vi "YOKOGAWA OPTIONS.vi"(8 "Error In":errorcluster, 11 "VISA resource name":refnum<visa-resource-name>) -> (0 "Error Out":errorcluster, 2 "Yokogawa Options":T1, 3 "VISA resource name out":refnum<visa-resource-name>)   [LabVIEW 2016]
uses:
  Type Definitions/YOKOGAWA Options.ctl
  <vilib>/Utility/error.llb/whitespace.ctl
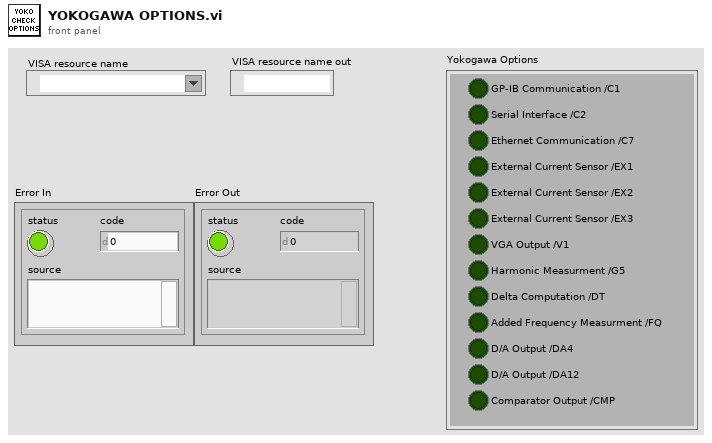
[diagram p1: front panel]
types:
  T1 = typedef "YOKOGAWA Options.ctl" = cluster{"GP-IB Communication /C1":bool, "Ethernet Communication /C7":bool, "External Current Sensor /EX1":bool, "External Current Sensor /EX2":bool, "External Current Sensor /EX3":bool, "VGA Output /V1":bool, "Harmonic Measurment /G5":bool, "Delta Computation /DT":bool, "Added Frequency Measurment /FQ":bool, "Serial Interface /C2":bool, "D/A Output /DA4":bool, "D/A Output /DA12":bool, "Comparator Output /CMP":bool}
  T2 = typedef "whitespace.ctl" = u16
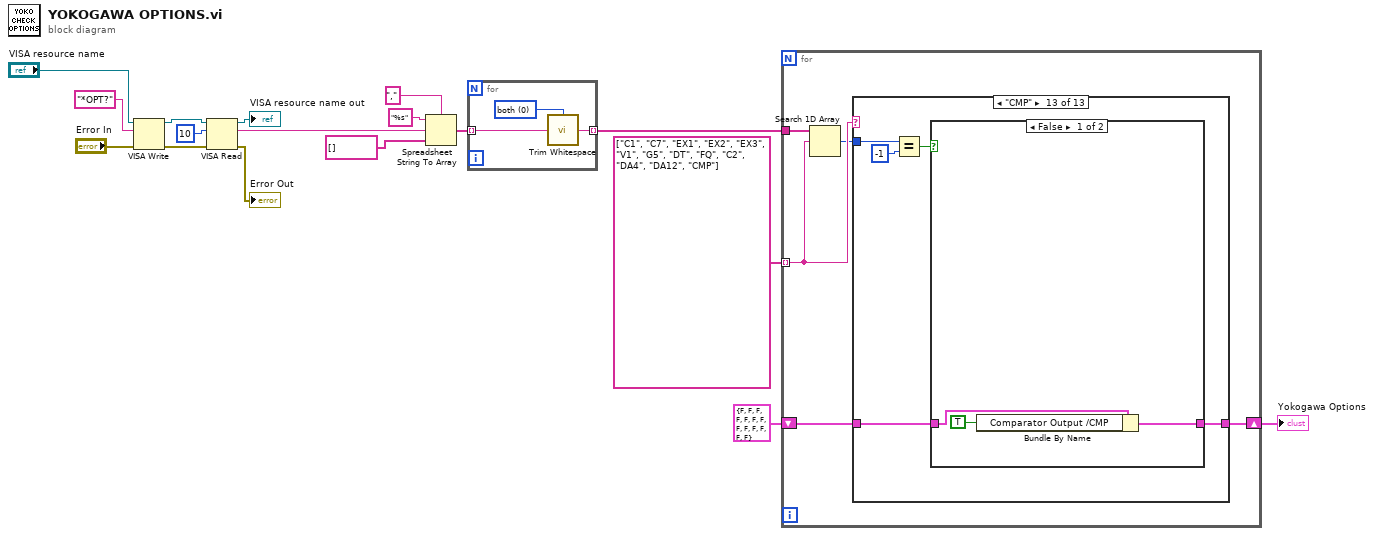
[diagram p0: block diagram]
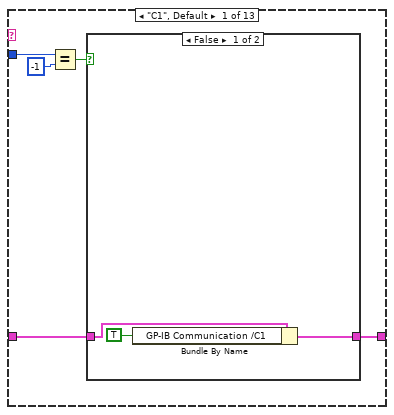
[diagram p2: hidden frame]
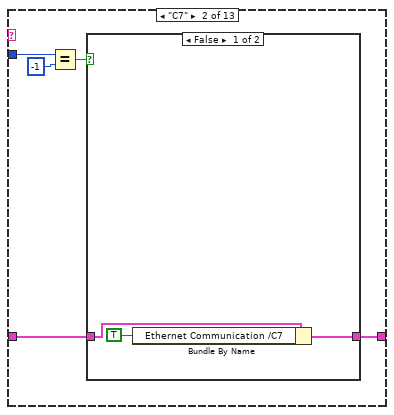
[diagram p4: hidden frame]
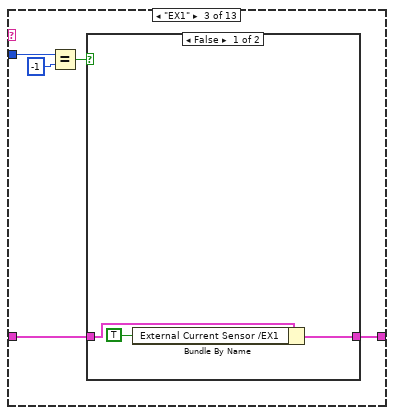
[diagram p6: hidden frame]
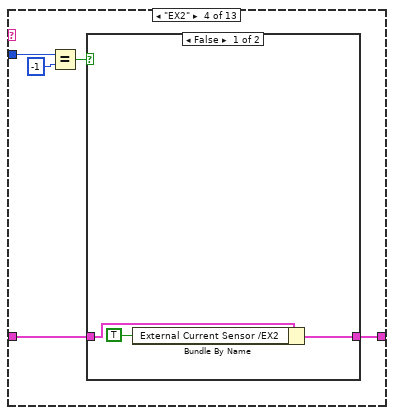
[diagram p8: hidden frame]
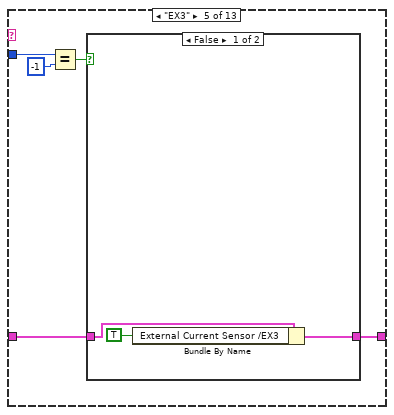
[diagram p10: hidden frame]
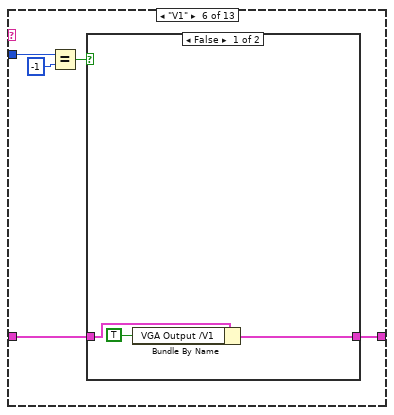
[diagram p12: hidden frame]
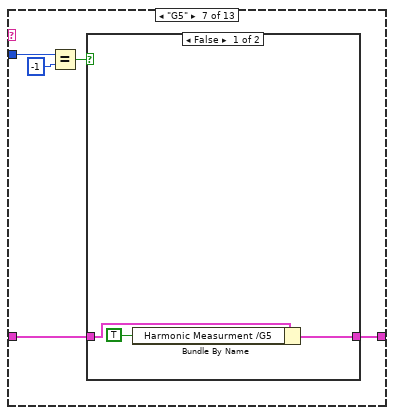
[diagram p14: hidden frame]
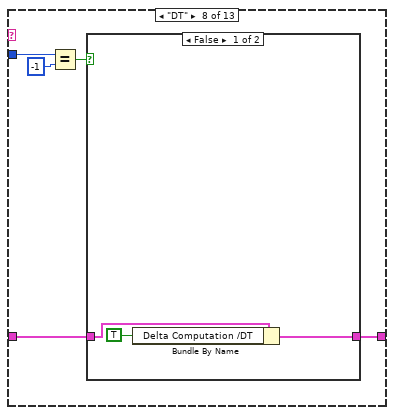
[diagram p16: hidden frame]
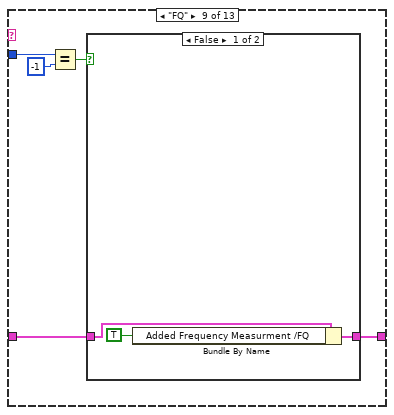
[diagram p18: hidden frame]
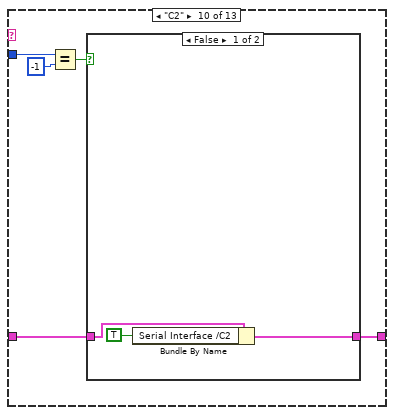
[diagram p20: hidden frame]
diagram:
  n1 = VISA Write(VISA resource name="VISA resource name", write buffer="*OPT?", error in (no error)="Error In") -> (VISA resource name out=w15:refnum<visa-resource-name>, error out=w13:errorcluster)  [unwired: 1 out]
  n2 = VISA Read(VISA resource name=w15, byte count=u32 10, error in (no error)=w13) -> (VISA resource name out=→"VISA resource name out":refnum<visa-resource-name>, read buffer=w11:string, error out=→"Error Out":errorcluster)  [unwired: 1 out]
  n3 = Spreadsheet String To Array(delimiter (Tab)=",", format string="%s", spreadsheet string=w11, array type (2D Dbl)=string[] []) -> (array=w7:string[])
  n4 = for {
    tunnel: w7 -> [w20] mode=indexing
    tunnel: [w18] -> w6 mode=indexing
    w19 = T2 0 items=["both", "start of string", "end of string"] ("location (both)")
    n5 = call <vilib>:"Trim Whitespace.vi"("string"=w20, "location (both)"=w19) -> ("trimmed string"=w18:string)
  }
  n6 = for {
    tunnel: w6 -> [w25]
    tunnel: string[] ["C1", "C7", "EX1", "EX2", "EX3", "V1", "G5", "DT", "FQ", "C2", "DA4", "DA12", "CMP"] -> [w24] mode=indexing
    shift-right: [w22] -> w3
    shift-left: T1 {"GP-IB Communication /C1"=FALSE, "Ethernet Communication /C7"=FALSE, "External Current Sensor /EX1"=FALSE, "External Current Sensor /EX2"=FALSE, "External Current Sensor /EX3"=FALSE, "VGA Output /V1"=FALSE, "Harmonic Measurment /G5"=FALSE, "Delta Computation /DT"=FALSE, "Added Frequency Measurment /FQ"=FALSE, "Serial Interface /C2"=FALSE, "D/A Output /DA4"=FALSE, "D/A Output /DA12"=FALSE, "Comparator Output /CMP"=FALSE} ("Yokogawa Options") -> [w23]
    n7 = Search 1D Array(1D array=w25, element=w24) -> (index of element=w21:i32)  [unwired: 1 in]
    n8 = case shown="\"CMP\"" w24 {
      tunnel: w23 -> [w27 w36 w45 w55 w64 w73 w82 w91 w100 w109 w118 w127 w136]
      tunnel: [w26 w37 w44 w53 w62 w72 w81 w89 w99 w108 w117 w126 w135] -> w22
      tunnel: w21 -> [w30 w35 w46 w54 w63 w71 w80 w90 w98 w107 w116 w125 w134]
      frame "C1", Default {
        n9 = Equal?(x=w30, y=-1) -> (x = y?=w28:bool)
        n10 = case shown="False" w28 {
          tunnel: w27 -> [w33 w34]
          tunnel: [w32 w34] -> w26
          frame False {
            n11 = Bundle By Name(cluster=w33, "GP-IB Communication /C1"=TRUE) -> (w32:T1)
          }
          frame True {
          }
        }
      }
      frame "C7" {
        n12 = Equal?(x=w35, y=-1) -> (x = y?=w38:bool)
        n13 = case shown="False" w38 {
          tunnel: w36 -> [w42 w43]
          tunnel: [w41 w43] -> w37
          frame False {
            n14 = Bundle By Name(cluster=w42, "Ethernet Communication /C7"=TRUE ("GP-IB Communication /C1")) -> (w41:T1)
          }
          frame True {
          }
        }
      }
      frame "EX1" {
        n15 = Equal?(x=w46, y=-1) -> (x = y?=w47:bool)
        n16 = case shown="False" w47 {
          tunnel: w45 -> [w51 w52]
          tunnel: [w50 w52] -> w44
          frame False {
            n17 = Bundle By Name(cluster=w51, "External Current Sensor /EX1"=TRUE ("GP-IB Communication /C1")) -> (w50:T1)
          }
          frame True {
          }
        }
      }
      frame "EX2" {
        n18 = Equal?(x=w54, y=-1) -> (x = y?=w56:bool)
        n19 = case shown="False" w56 {
          tunnel: w55 -> [w60 w61]
          tunnel: [w59 w61] -> w53
          frame False {
            n20 = Bundle By Name(cluster=w60, "External Current Sensor /EX2"=TRUE ("GP-IB Communication /C1")) -> (w59:T1)
          }
          frame True {
          }
        }
      }
      frame "EX3" {
        n21 = Equal?(x=w63, y=-1) -> (x = y?=w65:bool)
        n22 = case shown="False" w65 {
          tunnel: w64 -> [w69 w70]
          tunnel: [w68 w70] -> w62
          frame False {
            n23 = Bundle By Name(cluster=w69, "External Current Sensor /EX3"=TRUE ("GP-IB Communication /C1")) -> (w68:T1)
          }
          frame True {
          }
        }
      }
      frame "V1" {
        n24 = Equal?(x=w71, y=-1) -> (x = y?=w74:bool)
        n25 = case shown="False" w74 {
          tunnel: w73 -> [w78 w79]
          tunnel: [w77 w79] -> w72
          frame False {
            n26 = Bundle By Name(cluster=w78, "VGA Output /V1"=TRUE ("GP-IB Communication /C1")) -> (w77:T1)
          }
          frame True {
          }
        }
      }
      frame "G5" {
        n27 = Equal?(x=w80, y=-1) -> (x = y?=w83:bool)
        n28 = case shown="False" w83 {
          tunnel: w82 -> [w87 w88]
          tunnel: [w86 w88] -> w81
          frame False {
            n29 = Bundle By Name(cluster=w87, "Harmonic Measurment /G5"=TRUE ("GP-IB Communication /C1")) -> (w86:T1)
          }
          frame True {
          }
        }
      }
      frame "DT" {
        n30 = Equal?(x=w90, y=-1) -> (x = y?=w92:bool)
        n31 = case shown="False" w92 {
          tunnel: w91 -> [w96 w97]
          tunnel: [w95 w97] -> w89
          frame False {
            n32 = Bundle By Name(cluster=w96, "Delta Computation /DT"=TRUE ("GP-IB Communication /C1")) -> (w95:T1)
          }
          frame True {
          }
        }
      }
      frame "FQ" {
        n33 = Equal?(x=w98, y=-1) -> (x = y?=w101:bool)
        n34 = case shown="False" w101 {
          tunnel: w100 -> [w105 w106]
          tunnel: [w104 w106] -> w99
          frame False {
            n35 = Bundle By Name(cluster=w105, "Added Frequency Measurment /FQ"=TRUE ("GP-IB Communication /C1")) -> (w104:T1)
          }
          frame True {
          }
        }
      }
      frame "C2" {
        n36 = Equal?(x=w107, y=-1) -> (x = y?=w110:bool)
        n37 = case shown="False" w110 {
          tunnel: w109 -> [w114 w115]
          tunnel: [w113 w115] -> w108
          frame False {
            n38 = Bundle By Name(cluster=w114, "Serial Interface /C2"=TRUE ("GP-IB Communication /C1")) -> (w113:T1)
          }
          frame True {
          }
        }
      }
      frame "DA4" {
        n39 = Equal?(x=w116, y=-1) -> (x = y?=w119:bool)
        n40 = case shown="False" w119 {
          tunnel: w118 -> [w123 w124]
          tunnel: [w122 w124] -> w117
          frame False {
            n41 = Bundle By Name(cluster=w123, "D/A Output /DA4"=TRUE ("GP-IB Communication /C1")) -> (w122:T1)
          }
          frame True {
          }
        }
      }
      frame "DA12" {
        n42 = Equal?(x=w125, y=-1) -> (x = y?=w128:bool)
        n43 = case shown="False" w128 {
          tunnel: w127 -> [w132 w133]
          tunnel: [w131 w133] -> w126
          frame False {
            n44 = Bundle By Name(cluster=w132, "D/A Output /DA12"=TRUE ("GP-IB Communication /C1")) -> (w131:T1)
          }
          frame True {
          }
        }
      }
      frame "CMP" {
        n45 = Equal?(x=w134, y=-1) -> (x = y?=w137:bool)
        n46 = case shown="False" w137 {
          tunnel: w136 -> [w141 w142]
          tunnel: [w140 w142] -> w135
          frame False {
            n47 = Bundle By Name(cluster=w141, "Comparator Output /CMP"=TRUE ("GP-IB Communication /C1")) -> (w140:T1)
          }
          frame True {
          }
        }
      }
    }
  }
  "Yokogawa Options" <- w3
